vi "Set Default Channel Values.vi"(8 "error in (no error)":errorcluster, 9 "Values":dbl[](array[numeric]), 10 "Channels":string[](array[string]), 11 "SysDef Path":path) -> (0 "error out":errorcluster)   [LabVIEW 2015]
uses:
  NationalInstruments.VeriStand.SystemDefinitionAPI
  NationalInstruments.VeriStand.SystemStorage
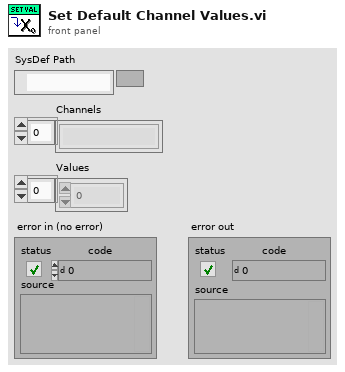
[diagram p1: front panel]
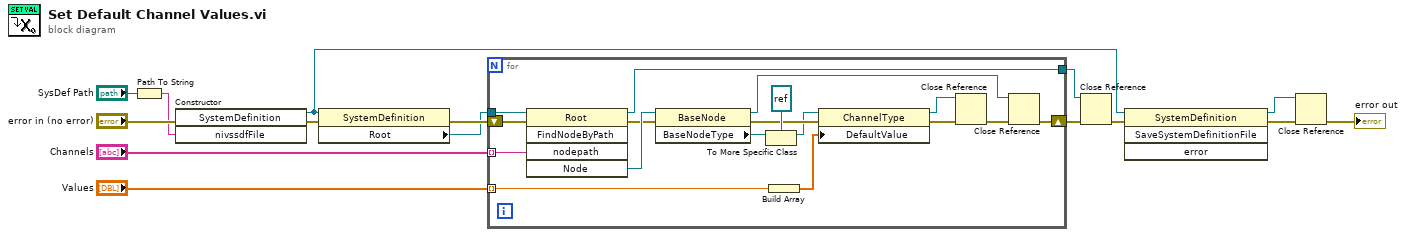
[diagram p0: block diagram]
diagram:
  n1 = Path To String(path="SysDef Path") -> (string=w12:string)
  n2 = constructor class="SystemDefinition"(error in="error in (no error)", "nivssdfFile"=w12) -> (reference out=w5:refnum<k24>, error out=w15:errorcluster)  [unwired: 2 in, 2 out]
  n3 = property class="SystemDefinition"(reference=w5, error in=w15) -> (error out=w11:errorcluster, "Root"=w9:refnum<k24>)  [unwired: 1 out]
  n4 = for {
    tunnel: w9 -> [w32]
    shift-right: [w19] -> w7
    shift-left: w11 -> [w31]
    tunnel: "Channels" -> [w29] mode=indexing
    tunnel: "Values" -> [w23] mode=indexing
    tunnel: [w16] -> w6
    n5 = invoke class="Root" method="FindNodeByPath"(reference=w32, error in=w31, "nodepath"=w29) -> (reference out=w16:refnum<k24>, error out=w28:errorcluster, "Node"=w30:refnum<k24>)  [unwired: 2 in, 2 out]
    n6 = property class="BaseNode"(reference=w30, error in=w28) -> (reference out=w17:refnum<k24>, error out=w25:errorcluster, "BaseNodeType"=w27:refnum<k24>)
    n7 = To More Specific Class(target class=refnum<k24> refnum ("reference out"), reference=w27) -> (specific class reference=w24:refnum<k24>)  [unwired: 1 in, 1 out]
    n8 = Build Array(w23) -> (w22:dbl[])
    n9 = property class="ChannelType"(reference=w24, error in=w25, "DefaultValue"=w22) -> (reference out=w18:refnum<k24>, error out=w21:errorcluster)
    n10 = Close Reference(reference=w18, error in (no error)=w21) -> (error out=w20:errorcluster)
    n11 = Close Reference(reference=w17, error in (no error)=w20) -> (error out=w19:errorcluster)
  }
  n12 = Close Reference(reference=w6, error in (no error)=w7) -> (error out=w4:errorcluster)
  n13 = invoke class="SystemDefinition" method="SaveSystemDefinitionFile"(reference=w5, error in=w4) -> (reference out=w2:refnum<k24>, error out=w3:errorcluster)  [unwired: 2 in, 2 out]
  n14 = Close Reference(reference=w2, error in (no error)=w3) -> (error out=→"error out":errorcluster)
